vi "Read Rotation (incremental).vi"(8 "error in (no error)":errorcluster, 11 "Gyro bias":cluster{"X":dbl, "Y":dbl, "Z":dbl}) -> (0 "error out":errorcluster, 3 "Angle":cluster{"X":dbl, "Y":dbl, "Z":dbl})   [LabVIEW 2017]
uses:
  <vilib>/Analysis/coordinate.llb/Angle Range (Degree).ctl
  <vilib>/Analysis/coordinate.llb/Angle Units.ctl
  <vilib>/Analysis/coordinate.llb/Wrap Angle (scalar).vi
  Globals/Gyro.vi
  MPU6050 Read Rotation Data.vi
  Calculate Orientation.vi
  <vilib>/Analysis/NI_AAL_Angle.lvlib
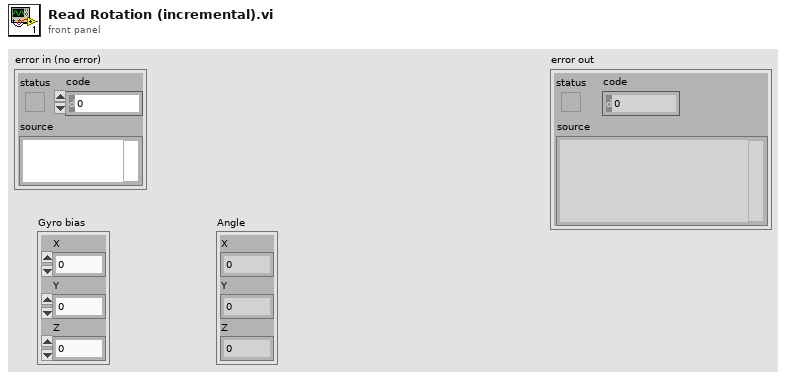
[diagram p1: front panel]
types:
  T1 = typedef "NI_AAL_Angle.lvlib/Angle Units.ctl" = i32
  T2 = typedef "NI_AAL_Angle.lvlib/Angle Range (Degree).ctl" = u16
  T3 = typedef "I2C.lvlib/I2C Reference.ctl" = cluster{"myRIO Reference":T4, "I2C Channels Enum":T8, "I2C Configuration":T9}
  T4 = typedef "myRIO Generic Hardware Reference.ctl" = cluster{"myRIO Model":T5, "myRIO Hardware Reference":T6}
  T5 = typedef "Hardware Version Enum.ctl" = enum16{"Unknown", "myRIO-1900", "myRIO-1950", "roboRIO", "NI ELVIS RIO CM"}
  T6 = typedef "myRIO v1.0 Reference.ctl" = cluster{"Generic FPGA Reference":T7, "Allow multiple opens":bool}
  T7 = typedef "Generic FPGA Reference.ctl" = refnum<k20>
  T8 = typedef "I2C Channels Enum.ctl" = enum16{"Not Connected", "A/I2C", "B/I2C", "I2C/I2C"}
  T9 = typedef "I2C.lvlib/I2C Configuration.ctl" = cluster{"I2C Transfer Rate":T10}
  T10 = typedef "I2C.lvlib/I2C Transfer Rate.ctl" = enum16{"Standard mode (100 kbps)", "Fast mode (400 kbps)"}
  T11 = cluster{"angle out":dbl, "angle out":dbl, "angle out":dbl}
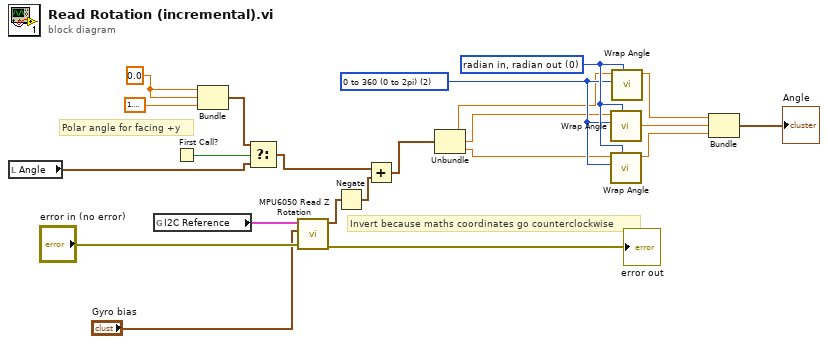
[diagram p0: block diagram]
diagram:
  w12 = 0.0
  w10 = T1 0 items=["radian in, radian out", "radian in, degree out", "degree in, degree out", "degree in, radian out"] ("angle units")
  w9 = T2 2 items=["none", "-180 to 180 (-pi to pi)", "0 to 360 (0 to 2pi)"] ("angle range")
  # "Invert because maths coordinates go counterclockwise"
  # "Polar angle for facing +y"
  n1 = local read "Angle"() -> (w18:cluster{"X":dbl, "Y":dbl, "Z":dbl})
  n2 = global read "Gyro.vi" "I2C Reference"() -> (w22:T3)
  n3 = First Call?() -> (First Call?: T/F=w19:bool)
  n4 = Bundle(w12, w12, 1.5707963267948966) -> (w11:cluster{dbl, dbl, dbl})  [unwired: 1 in]
  n5 = Select(t=w11, s=w19, f=w18) -> (s? t:f=w17:cluster{"X":dbl, "Y":dbl, "Z":dbl})
  n6 = call "MPU6050 Read Z Rotation.vi"("error in (no error)"="error in (no error)", "Gyro bias"="Gyro bias", "I2C Ref In"=w22) -> ("error out"=→"error out":errorcluster, "Total Rotation (rads)"=w15:cluster{"X":dbl, "Y":dbl, "Z":dbl})  [unwired: 7 in]
  n7 = Negate(x=w15) -> (-x=w16:cluster{"X":dbl, "Y":dbl, "Z":dbl})
  n8 = Add(x=w17, y=w16) -> (x+y=w8:cluster{"X":dbl, "Y":dbl, "Z":dbl})
  n9 = Unbundle(w8) -> ("X"=w1:dbl, "Y"=w2:dbl, "Z"=w3:dbl)
  n10 = call-poly <vilib>:"Wrap Angle.vi"("angle units"=w10, "angle range"=w9, "angle in"=w2) -> ("angle out"=w6:dbl)  [unwired: 7 in, 1 out]
  n11 = call-poly <vilib>:"Wrap Angle.vi"("angle units"=w10, "angle range"=w9, "angle in"=w3) -> ("angle out"=w5:dbl)  [unwired: 7 in, 1 out]
  n12 = call-poly <vilib>:"Wrap Angle.vi"("angle units"=w10, "angle range"=w9, "angle in"=w1) -> ("angle out"=w7:dbl)  [unwired: 7 in, 1 out]
  n13 = Bundle("angle out"=w7, "angle out"=w6, "angle out"=w5) -> (→"Angle":T11)  [unwired: 1 in]
